vi "RT Driver VI.vi"(7 "Operation":T1, 11 "Device Reference in":T2 format="%.0x") -> (0 "Error Code":i32)   [LabVIEW 2026, in "Runtime Configuration Support Inline Async Example Custom Device Engine.lvlib"]
uses:
  Runtime Configuration Support Inline Async Example Custom Device Engine.lvlib
  <vilib>/NI VeriStand/Custom Device API/Custom Device Item Ref.ctl
  <vilib>/NI VeriStand/Custom Device API/Hardware Interface Driver VI Operation.ctl
  Shared/Compiled.Settings.ctl
  <vilib>/NI/NIVS Inline Async API/_VS Inline Async API/VS Inline Async API/VS Inline Async API.lvclass
  Parameter.ctl
  AsyncRequest.ctl
  Shared/Reconfigured.Settings.ctl
  <vilib>/NI VeriStand/Custom Device API/Block Data Reference.ctl
  <vilib>/NI VeriStand/Custom Device API/Data Reference.ctl
  <vilib>/NI/NIVS Inline Async API/_VS Inline Async API/VS Inline Async API/VS Inline Async API.lvclass/VS Inline Async API.ctl
  <vilib>/NI/NIVS Inline Async API/_Data Access Engine/Data Access Engine/Data Access Engine.lvclass/Data Access Engine.ctl
  <vilib>/NI/NIVS Inline Async API/_Data Access Engine/Access Type Classes/Write/Write.lvclass/Write.ctl
  <vilib>/NI/NIVS Inline Async API/_Data Access Engine/Access Type Classes/ReadWrite/ReadWrite.lvclass/ReadWrite.ctl
  <vilib>/NI/NIVS Inline Async API/_Data Access Engine/Access Type Classes/Read/Read.lvclass/Read.ctl
  <vilib>/NI/NIVS Inline Async API/_Data Access Engine/Data Access Engine/Methods/Data.Engine.Read Data from HW.vi
  <vilib>/NI/NIVS Inline Async API/_VS Inline Async API/Error Handling Process/SubVIs/Error.GetError.vi
  <vilib>/NI/NIVS Inline Async API/_Data Access Engine/Data Access Engine/Methods/Data.Engine.Write Data to HW.vi
  <vilib>/NI/NIVS Inline Async API/_Data Access Engine/Access Type Classes/ReadWrite/ReadWrite.EngineData.vi
  <vilib>/NI/NIVS Inline Async API/_Data Access Engine/Access Type Classes/Write/Write.EngineData.vi
  <vilib>/NI/NIVS Inline Async API/_Data Access Engine/Access Type Classes/Read/Read.EngineData.vi
  <vilib>/NI VeriStand/Custom Device API/NI VeriStand - Get Channel Value by Data Reference.vi
  <vilib>/NI VeriStand/Custom Device API/NI VeriStand - Set Channel Value by Data Reference.vi
  <vilib>/NI VeriStand/Custom Device API/NI VeriStand - Set Channel Values by Block Data Reference.vi
  <vilib>/NI VeriStand/Custom Device API/NI VeriStand - Get Channel Values by Block Data Reference.vi
  Runtime Configuration Support Inline Async Example Custom Device.Async.vi
  Shared/Constants.vi
  Command Loop.vi
  <vilib>/NI VeriStand/Custom Device API/Get Item Property (Variant).vi
  <vilib>/NI VeriStand/Custom Device API/Global Data Refs.vi
  <vilib>/NI/NIVS Inline Async API/_Data Access Engine/Data Access Engine/Data Access Engine.lvclass
  Shared/Runtime Configuration Support Inline Async Example Custom Device Shared.lvlib
  <vilib>/NI VeriStand/Custom Device Tools/Custom Device Utility Library/Custom Device Utility Library.lvlib
  <vilib>/NI VeriStand/Custom Device API/Custom Device API.lvlib
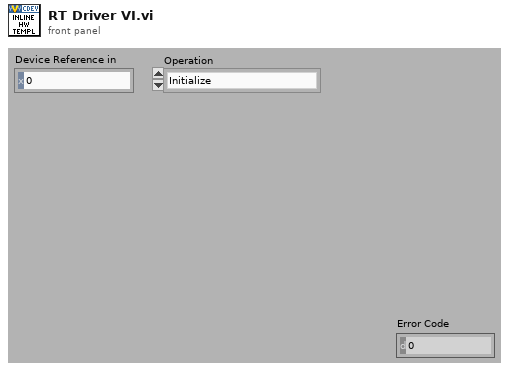
[diagram p1: front panel]
types:
  T1 = typedef "Custom Device API.lvlib/Hardware Interface Driver VI Operation.ctl" = enum16{"Initialize", "Start", "Read Data from HW", "Write Data to HW", "Close"}
  T2 = typedef "Custom Device API.lvlib/Custom Device Item Ref.ctl" = u64
  T3 = typedef "Runtime Configuration Support Inline Async Example Custom Device Engine.lvlib/Parameter.ctl" = cluster{"Compiled.Settings":T4, "Async Request Ref":refnum<queue>}
  T4 = typedef "Runtime Configuration Support Inline Async Example Custom Device Shared.lvlib/Compiled.Settings.ctl" = cluster{"Name":string, "Async Init Timeout":u16, "Inport SignalIDs":i32[], "Outport SignalIDs":i32[], "Inport Values":dbl[], "Outport Values":dbl[], "Dynamic Config Status":bool, "Device Error":errorcluster}
  T5 = typedef "Runtime Configuration Support Inline Async Example Custom Device Shared.lvlib/Reconfigured.Settings.ctl" = cluster{"Compiled.Settings":T4, "Compiled Inline Async Settings":cluster{"Read":cluster{"Refs":T6[], "Values":dbl[]}[], "Write":cluster{"Refs":T6[], "Values":dbl[]}[], "ReadWrite":cluster{"Refs":T7[], "Values":dbl[], "Reset Values":dbl[]}[], "LUT":variant}, "Response Ref":refnum<queue>}
  T6 = typedef "Custom Device API.lvlib/Block Data Reference.ctl" = cluster{"Data Reference":T7, "Offset":u64, "Length":u64}
  T7 = typedef "Custom Device API.lvlib/Data Reference.ctl" = i32
  T8 = cluster{"Async":refnum<class "VS Inline Async API.lvclass">, "Parameter":T3, "ReConfigured.Settings":T5}
  T9 = cluster{"Reconfigured.Settings Ref":refnum<queue>}
  T10 = typedef "Runtime Configuration Support Inline Async Example Custom Device Engine.lvlib/AsyncRequest.ctl" = cluster{"Compiled.Settings":T4, "Data Access":variant, "Async Response Ref":refnum<queue>}
  T11 = cluster{"Dynamic Config Status":bool, "Error":errorcluster}
  T12 = cluster{"Read":cluster{"Refs":T6[], "Values":dbl[]}[], "Write":cluster{"Refs":T6[], "Values":dbl[]}[], "ReadWrite":cluster{"Refs":T7[], "Values":dbl[], "Reset Values":dbl[]}[], "LUT":variant}
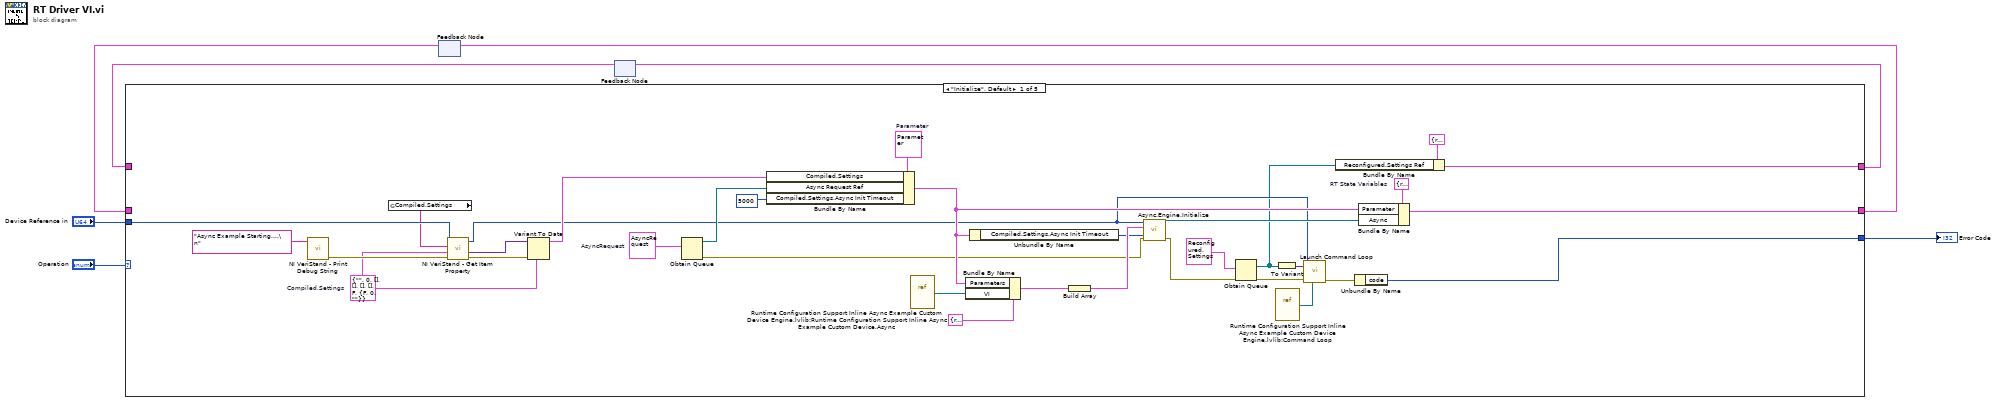
[diagram p0: block diagram]
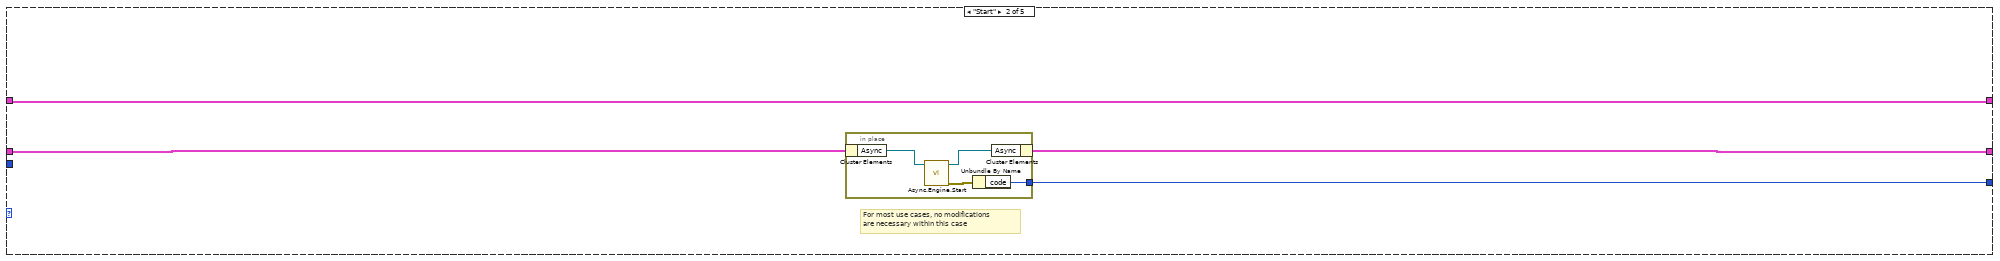
[diagram p2: hidden frame]
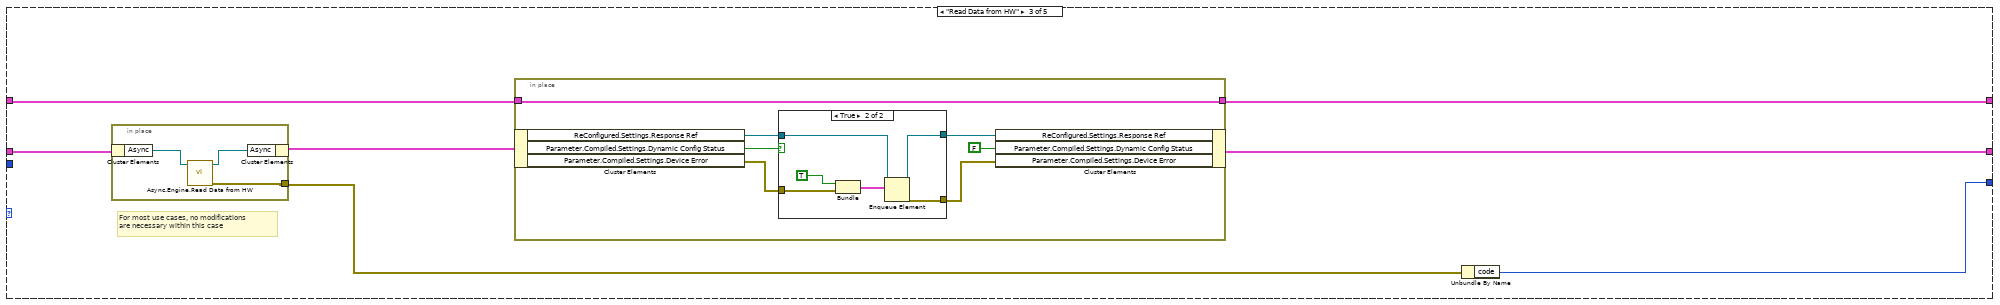
[diagram p3: hidden frame]
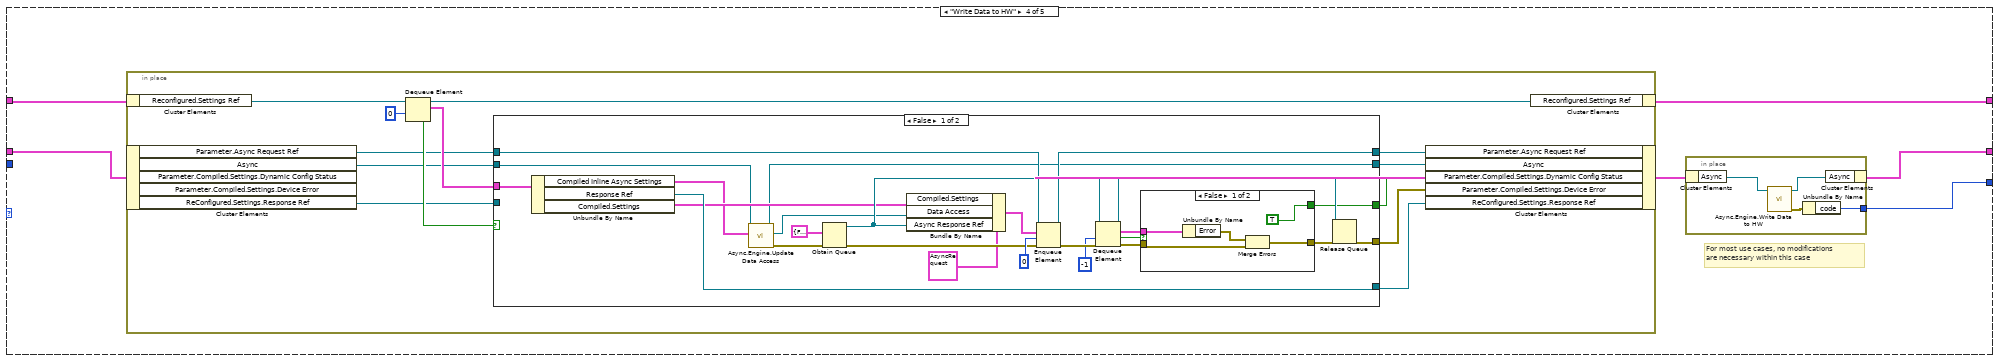
[diagram p5: hidden frame]
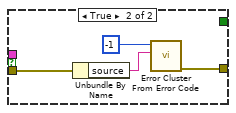
[diagram p6: hidden frame]
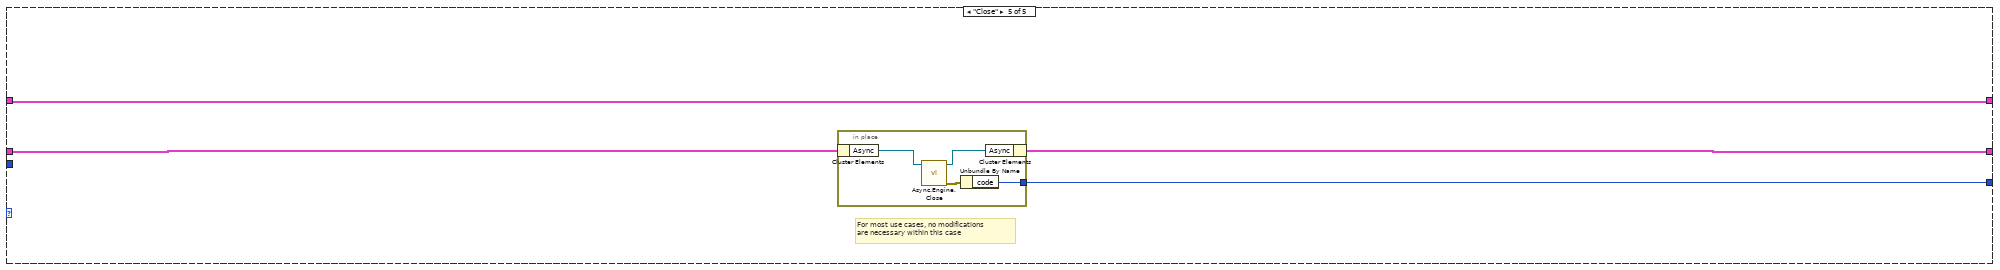
[diagram p8: hidden frame]
diagram:
  n1 = feedback #1() -> (w5:T8)  [unwired: 1 out]
  n2 = feedback #2() -> (w1:T9)  [unwired: 1 in]
  n3 = case shown="\"Initialize\", Default" "Operation" {
    tunnel: [w38 w43 w53 w78 w136] -> w6
    tunnel: w5 -> [_ w44 w55 w74 w137]
    tunnel: "Device Reference in" -> [w29 _ _ _ _]
    tunnel: [w40 w42 w51 w79 w135] -> w3
    tunnel: [w9 w41 w50 w76 w134] -> w2
    tunnel: w1 -> [_ w41 w49 w77 w134]
    frame "Initialize", Default {
      w24 = T10 {"Compiled.Settings"={"Name"="", "Async Init Timeout"=0, "Inport SignalIDs"=[], "Outport SignalIDs"=[], "Inport Values"=[], "Outport Values"=[], "Dynamic Config Status"=FALSE, "Device Error"={"status"=FALSE, "code"=0, "source"=""}}, "Data Access"=variant(u16 0), "Async Response Ref"=refnum}  # AsyncRequest
      w21 = T3 {"Compiled.Settings"={"Name"="", "Async Init Timeout"=0, "Inport SignalIDs"=[], "Outport SignalIDs"=[], "Inport Values"=[], "Outport Values"=[], "Dynamic Config Status"=FALSE, "Device Error"={"status"=FALSE, "code"=0, "source"=""}}, "Async Request Ref"=refnum}  # Parameter
      w35 = T8 {"Async"=refnum, "Parameter"={"Compiled.Settings"={"Name"="", "Async Init Timeout"=0, "Inport SignalIDs"=[], "Outport SignalIDs"=[], "Inport Values"=[], "Outport Values"=[], "Dynamic Config Status"=FALSE, "Device Error"={"status"=FALSE, "code"=0, "source"=""}}, "Async Request Ref"=refnum}, "ReConfigured.Settings"={"Compiled.Settings"={"Name"="", "Async Init Timeout"=0, "Inport SignalIDs"=[], "Outport SignalIDs"=[], "Inport Values"=[], "Outport Values"=[], "Dynamic Config Status"=FALSE, "Device Error"={"status"=FALSE, "code"=0, "source"=""}}, "Compiled Inline Async Settings"={"Read"=[], "Write"=[], "ReadWrite"=[], "LUT"=variant}, "Response Ref"=refnum}}  # RT State Variables
      w18 = T4 {"Name"="", "Async Init Timeout"=0, "Inport SignalIDs"=[], "Outport SignalIDs"=[], "Inport Values"=[], "Outport Values"=[], "Dynamic Config Status"=FALSE, "Device Error"={"status"=FALSE, "code"=0, "source"=""}}  # Compiled.Settings
      n4 = call <vilib>:"NI VeriStand - Print Debug String.vi"("Message"="Async Example Starting....\n") -> ("error out"=w31:errorcluster)  [unwired: 10 in]
      n5 = global read "Constants.vi" "Compiled.Settings"() -> (w27:string)
      n6 = call-poly <vilib>:"NI VeriStand - Get Item Property.vi"("error in (no error)"=w31, "Default Value"=w18, "Property Name"=w27, "Item Ref in"=w29) -> ("error out"=w26:errorcluster, "Value"=w28:variant, "Item Ref out"=w14:T2)  [unwired: 4 in, 1 out]
      n7 = Variant To Data(error in=w26, type=w18, Variant=w28) -> (data=w25:T4)  [unwired: 1 out]
      n8 = Obtain Queue(element data type=w24) -> (queue out=w23:refnum<queue>, error out=w19:errorcluster)  [unwired: 4 in, 1 out]
      n9 = Bundle By Name(cluster=w21, "Compiled.Settings"=w25, "Async Request Ref"=w23, "Compiled.Settings.Async Init Timeout"=u16 5000) -> (w22:T3)
      n10 = vi-ref "Runtime Configuration Support Inline Async Example Custom Device Engine.lvlib:Runtime Configuration Support Inline Async Example Custom Device.Async.vi"() -> (w32:refnum<vi>)
      n11 = Bundle By Name(cluster=cluster{"VI":refnum<vi>, "Parameters":variant} {"VI"=refnum, "Parameters"=variant} ("Process"), "Parameters"=w22, "VI"=w32) -> (w36:cluster{"VI":refnum<vi>, "Parameters":variant})
      n12 = Unbundle By Name(w22) -> ("Compiled.Settings.Async Init Timeout"=w30:u16)
      n13 = Build Array(w36) -> (w34:cluster{"VI":refnum<vi>, "Parameters":variant}[])
      n14 = call <vilib>:"Async.Engine.Initialize.vi"("Timeout (ms) (5000)"=w30, "error in (no error)"=w19, "Processes"=w34, "Custom Device Ref"=w14) -> ("error out"=w13:errorcluster, "Async"=w39:refnum<class "VS Inline Async API.lvclass">)  [unwired: 6 in]
      n15 = Obtain Queue(element data type=T5 {"Compiled.Settings"={"Name"="", "Async Init Timeout"=0, "Inport SignalIDs"=[], "Outport SignalIDs"=[], "Inport Values"=[], "Outport Values"=[], "Dynamic Config Status"=FALSE, "Device Error"={"status"=FALSE, "code"=0, "source"=""}}, "Compiled Inline Async Settings"={"Read"=[], "Write"=[], "ReadWrite"=[], "LUT"=variant}, "Response Ref"=refnum} ("Reconfigure.Settings.ctl"), error in (no error)=w13) -> (queue out=w8:refnum<queue>, error out=w12:errorcluster)  [unwired: 3 in, 1 out]
      n16 = vi-ref "Runtime Configuration Support Inline Async Example Custom Device Engine.lvlib:Command Loop.vi"() -> (w16:refnum<vi>)
      n17 = To Variant(anything=w8) -> (Variant=w17:variant)
      n18 = call "Launch Command Loop.vi"("VI Refnum"=w16, "error in"=w12, "Queue Refs"=w17, "Device Reference in"=w14) -> ("error out"=w15:errorcluster)  [unwired: 7 in]
      n19 = Bundle By Name(cluster=T9 {"Reconfigured.Settings Ref"=refnum} ("Queue Refs in"), "Reconfigured.Settings Ref"=w8) -> (w9:T9)
      n20 = Unbundle By Name(w15) -> ("code"=w40:i32)
      n21 = Bundle By Name(cluster=w35, "Parameter"=w22, "Async"=w39) -> (w38:T8)
    }
    frame "Start" {
      # "For most use cases, no modifications \nare necessary within this case"
      n22 = in-place {
        in-place-border: [w45] -> w42
        n23 = in-place-cluster #3(w44) -> ("Async"=w48:refnum<class "VS Inline Async API.lvclass">)
        n24 = call <vilib>:"Async.Engine.Start.vi"("VS Inline Async API in"=w48) -> ("error out"=w46:errorcluster, "VS Inline Async API out"=w47:refnum<class "VS Inline Async API.lvclass">)  [unwired: 9 in]
        n25 = Unbundle By Name(w46) -> ("code"=w45:i32)
        n26 = in-place-cluster #3("Async"=w47) -> (w43:T8)
      }
    }
    frame "Read Data from HW" {
      # "For most use cases, no modifications \nare necessary within this case"
      n27 = in-place {
        in-place-border: [w71] -> w52
        n28 = in-place-cluster #4(w55) -> ("Async"=w73:refnum<class "VS Inline Async API.lvclass">)
        n29 = call <vilib>:"Async.Engine.Read Data from HW.vi"("Async in"=w73) -> ("error out"=w71:errorcluster, "Async out"=w72:refnum<class "VS Inline Async API.lvclass">)  [unwired: 9 in]
        n30 = in-place-cluster #4("Async"=w72) -> (w54:T8)
      }
      n31 = in-place {
        in-place-border: [w56] -> w50
        in-place-border: w49 -> [w56]
        n32 = in-place-cluster #5(w54) -> ("ReConfigured.Settings.Response Ref"=w58:refnum<queue>, "Parameter.Compiled.Settings.Dynamic Config Status"=w62:bool, "Parameter.Compiled.Settings.Device Error"=w61:errorcluster)
        n33 = case shown="True" w62 {
          tunnel: [w63 w70] -> w57
          tunnel: w61 -> [w64 w68]
          tunnel: [w64 w65] -> w60
          tunnel: w58 -> [w63 w66]
          frame False {
          }
          frame True {
            n34 = Bundle(TRUE, "Device Error"=w68) -> (w67:cluster{bool, "Device Error":errorcluster})  [unwired: 1 in]
            n35 = Enqueue Element(queue=w66, element=w67) -> (queue out=w70:refnum<queue>, error out=w65:errorcluster)  [unwired: 2 in, 1 out]
          }
        }
        n36 = in-place-cluster #5("ReConfigured.Settings.Response Ref"=w57, "Parameter.Compiled.Settings.Dynamic Config Status"=FALSE ("Compiled.Settings.Compiled Info.Dynamic Config Status"), "Parameter.Compiled.Settings.Device Error"=w60) -> (w53:T8)
      }
      n37 = Unbundle By Name(w52) -> ("code"=w51:i32)
    }
    frame "Write Data to HW" {
      # "For most use cases, no modifications \nare necessary within this case"
      n38 = in-place {
        n39 = in-place-cluster #6(w77) -> ("Reconfigured.Settings Ref"=w81:refnum<queue>)
        n40 = in-place-cluster #7(w74) -> ("Parameter.Async Request Ref"=w89:refnum<queue>, "Async"=w87:refnum<class "VS Inline Async API.lvclass">, "ReConfigured.Settings.Response Ref"=w83:refnum<queue>)  [unwired: 2 out]
        n41 = Dequeue Element(queue=w81, timeout in ms (-1)=0) -> (queue out=w80:refnum<queue>, element=w90:T5, timed out?=w91:bool)  [unwired: 1 in, 1 out]
        n42 = case shown="False" w91 {
          tunnel: w90 -> [w114 _]
          tunnel: w89 -> [w115 w129]
          tunnel: [w116 w129] -> w88
          tunnel: w87 -> [w95 w128]
          tunnel: [w94 w128] -> w86
          tunnel: [w104 _] -> w84
          tunnel: [w102 _] -> w85
          tunnel: w83 -> [_ w127]
          tunnel: [w99 w127] -> w82
          frame False {
            n43 = Unbundle By Name(w114) -> ("Compiled Inline Async Settings"=w96:T12, "Response Ref"=w99:refnum<queue>, "Compiled.Settings"=w98:T4)
            n44 = call <vilib>:"Async.Engine.Update Data Access.vi"("Compiled.InlineAsync.Settings"=w96, "Async in"=w95) -> ("error out"=w97:errorcluster, "Data Access Engine"=w93:refnum<class "Data Access Engine.lvclass">, "Async out"=w94:refnum<class "VS Inline Async API.lvclass">)  [unwired: 7 in]
            n45 = Obtain Queue(element data type=T11 {"Dynamic Config Status"=FALSE, "Error"={"status"=FALSE, "code"=0, "source"=""}}, error in (no error)=w97) -> (queue out=w101:refnum<queue>, error out=w111:errorcluster)  [unwired: 3 in, 1 out]
            n46 = Bundle By Name(cluster=T10 {"Compiled.Settings"={"Name"="", "Async Init Timeout"=0, "Inport SignalIDs"=[], "Outport SignalIDs"=[], "Inport Values"=[], "Outport Values"=[], "Dynamic Config Status"=FALSE, "Device Error"={"status"=FALSE, "code"=0, "source"=""}}, "Data Access"=variant, "Async Response Ref"=refnum} ("AsyncRequest"), "Compiled.Settings"=w98, "Data Access"=w93, "Async Response Ref"=w101) -> (w112:T10)
            n47 = Enqueue Element(queue=w115, element=w112, timeout in ms (-1)=0, error in (no error)=w111) -> (queue out=w116:refnum<queue>, error out=w110:errorcluster)  [unwired: 1 out]
            n48 = Dequeue Element(queue=w101, timeout in ms (-1)=-1, error in (no error)=w110) -> (queue out=w105:refnum<queue>, element=w103:T11, timed out?=w108:bool, error out=w107:errorcluster)
            n49 = case shown="False" w108 {
              tunnel: w107 -> [w119 w125]
              tunnel: [w118 w123] -> w106
              tunnel: w103 -> [w121 _]
              tunnel: [TRUE ("Dynamic Config Status") _] -> w102
              frame False {
                n50 = Unbundle By Name(w121) -> ("Error"=w120:errorcluster)
                n51 = Merge Errors(w120, w119) -> (w118:errorcluster)
              }
              frame True {
                n52 = Unbundle By Name(w125) -> ("source"=w124:string)
                n53 = call <vilib>:"Error Cluster From Error Code.vi"("error message (\"\")"=w124, "error code (0)"=-1) -> ("error out"=w123:errorcluster)  [unwired: 7 in]
              }
            }
            n54 = Release Queue(queue=w105, error in (no error)=w106) -> (error out=w104:errorcluster)  [unwired: 1 in, 2 out]
          }
          frame True {
          }
        }
        n55 = in-place-cluster #7("Parameter.Async Request Ref"=w88, "Async"=w86, "Parameter.Compiled.Settings.Dynamic Config Status"=w85, "Parameter.Compiled.Settings.Device Error"=w84, "ReConfigured.Settings.Response Ref"=w82) -> (w75:T8)
        n56 = in-place-cluster #6("Reconfigured.Settings Ref"=w80) -> (w76:T9)
      }
      n57 = in-place {
        in-place-border: [w133] -> w79
        n58 = in-place-cluster #8(w75) -> ("Async"=w131:refnum<class "VS Inline Async API.lvclass">)
        n59 = call <vilib>:"Async.Engine.Write Data to HW.vi"("VS Inline Async API in"=w131) -> ("error out"=w132:errorcluster, "VS Inline Async API out"=w130:refnum<class "VS Inline Async API.lvclass">)  [unwired: 9 in]
        n60 = Unbundle By Name(w132) -> ("code"=w133:i32)
        n61 = in-place-cluster #8("Async"=w130) -> (w78:T8)
      }
    }
    frame "Close" {
      # "For most use cases, no modifications \nare necessary within this case"
      n62 = in-place {
        in-place-border: [w139] -> w135
        n63 = in-place-cluster #9(w137) -> ("Async"=w141:refnum<class "VS Inline Async API.lvclass">)
        n64 = call <vilib>:"Async.Engine.Close.vi"("Async in"=w141) -> ("error out"=w138:errorcluster, "Async out"=w140:refnum<class "VS Inline Async API.lvclass">)  [unwired: 9 in]
        n65 = Unbundle By Name(w138) -> ("code"=w139:i32)
        n66 = in-place-cluster #9("Async"=w140) -> (w136:T8)
      }
    }
  }
  "Error Code" <- w3
  n67 = feedback-in #1(w6) -> ()
  n68 = feedback-in #2(w2) -> ()
